vi "ENC_IO_Config.vi"(1 "dt":dbl=0.0005 min=0.0005 step=1e-05) -> (3 "AO Task":refnum<k21>, 4 "ENC Task":refnum<k21>, 5 "AI Task":refnum<k21>, 6 "IO error out":errorcluster)   [LabVIEW 2020]
panel:
  in  "IO Config":T1={"srv02 analog output"=0, "srv02 encoder"=0, "dev"="Dev1"}
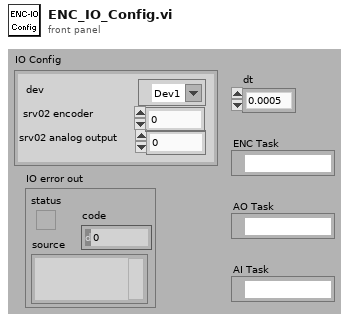
[diagram p1: front panel]
types:
  T1 = cluster{"srv02 analog output":u32, "srv02 encoder":u32, "dev":tag}
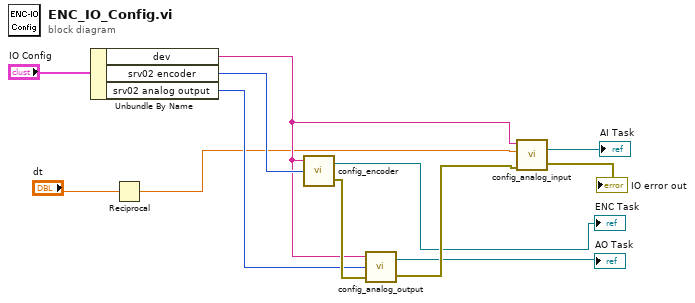
[diagram p0: block diagram]
diagram:
  n1 = Unbundle By Name("IO Config") -> ("dev"=w8:tag, "srv02 encoder"=w10:u32, "srv02 analog output"=w9:u32)
  n2 = Reciprocal(x="dt") -> (1/x=w6:dbl)
  n3 = call "config_encoder.vi"("encoder channel"=w10, "dev"=w8) -> ("error out"=w12:errorcluster, "task out"=→"ENC Task":refnum<k21>)  [unwired: 1 in]
  n4 = call "config_analog_output.vi"("error in"=w12, "analog output channel"=w9, "dev"=w8) -> ("error out"=w5:errorcluster, "task out"=→"AO Task":refnum<k21>)
  n5 = call "config_analog_input.vi"("dev"=w8, "sampling rate (Hz)"=w6, "error in"=w5) -> ("task out"=→"AI Task":refnum<k21>, "error out"=→"IO error out":errorcluster)  [unwired: 2 in]
